vi "Bridge Bias Get Capabilities.vi"(8 "error in":errorcluster, 11 "bridge in":T1={"type"=enum."TWM client", "TWM"={"pipe name"="", "parameters"=[], "handle"=0, "fixed aper [s]"=0.0, "f-list [Hz]"=[], "discrete f-list"=FALSE, "unc mode"=enum."None", "unc mcc"=0, "unc first"=FALSE}, "last f"=0.0, "bias comp"={"bias type"=enum."dummy", "VISA"="", "Enable"=FALSE, "channel qu"=[], "channel Uinit"=[]}, "sim mode"=enum."Generic RLC network", "channel idns"=[], "sim phases"=1} {"TWM"."f-list [Hz]" format="%#_6p"}) -> (0 "error out":errorcluster, 1 "channels count":i32, 2 "max. level [V]":dbl, 3 "bridge out":T1={"type"=enum."TWM client", "TWM"={"pipe name"="", "parameters"=[], "handle"=0, "fixed aper [s]"=0.0, "f-list [Hz]"=[], "discrete f-list"=FALSE, "unc mode"=enum."None", "unc mcc"=0, "unc first"=FALSE}, "last f"=0.0, "bias comp"={"bias type"=enum."dummy", "VISA"="", "Enable"=FALSE, "channel qu"=[], "channel Uinit"=[]}, "sim mode"=enum."Generic RLC network", "channel idns"=[], "sim phases"=1} {"TWM"."f-list [Hz]" format="%#_6p"})   [LabVIEW 2020]
doc: "Get basic capabilities of DC bias compensator."
uses:
  Bridge Session.ctl
  Bridge Type.ctl
  drivers/TWM client/TWM Session.ctl
  drivers/TWM client/TWM parameters.ctl
  drivers/TWM client/Meas Proc QWTB Uncertainty Mode.ctl
  Bridge Bias Session.ctl
  Bridge Bias Type.ctl
  Bridge Sim Mode.ctl
  <vilib>/Utility/error.llb/Error Cluster From Error Code.vi
  <vilib>/ErrorRing/Error Ring.xnode
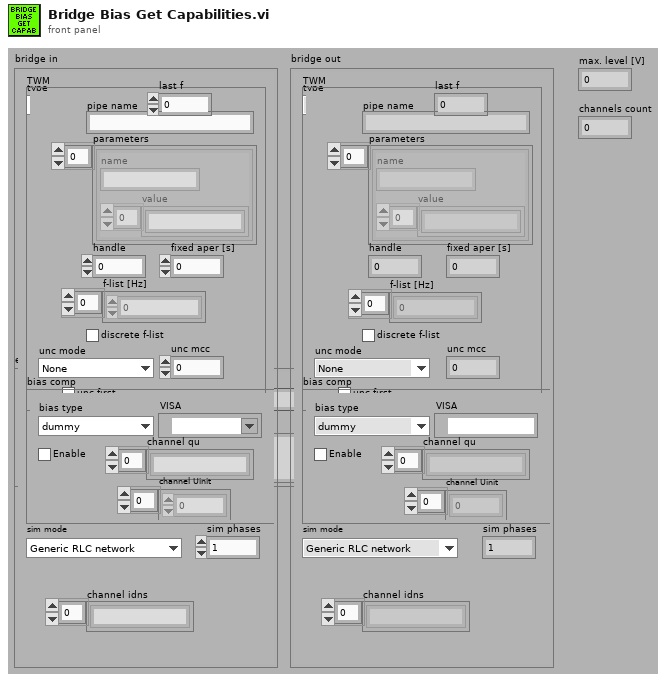
[diagram p1: front panel]
types:
  T1 = typedef "Bridge Session.ctl" = cluster{"type":T2, "TWM":T3, "last f":dbl, "bias comp":T6, "sim mode":T8, "channel idns":string[], "sim phases":i32}
  T2 = typedef "Bridge Type.ctl" = enum16{"TWM client", "dummy"}
  T3 = typedef "TWM Session.ctl" = cluster{"pipe name":string, "parameters":T4[], "handle":i32, "fixed aper [s]":dbl, "f-list [Hz]":dbl[], "discrete f-list":bool, "unc mode":T5, "unc mcc":i32, "unc first":bool}
  T4 = typedef "TWM parameters.ctl" = cluster{"name":string, "value":string[]}
  T5 = typedef "Meas Proc QWTB Uncertainty Mode.ctl" = enum16{"None", "GUF", "Monte Carlo"}
  T6 = typedef "Bridge Bias Session.ctl" = cluster{"bias type":T7, "VISA":refnum<visa-resource-name>, "Enable":bool, "channel qu":string[], "channel Uinit":dbl[]}
  T7 = typedef "Bridge Bias Type.ctl" = enum16{"dummy", "CMI LiBbias V1.0"}
  T8 = typedef "Bridge Sim Mode.ctl" = enum16{"Generic RLC network", "Interchannel transfer"}
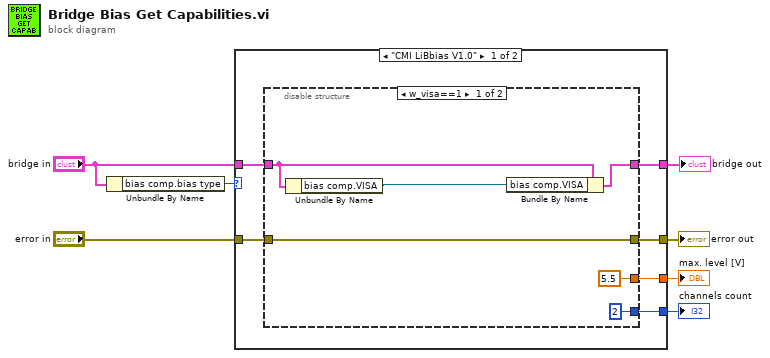
[diagram p0: block diagram]
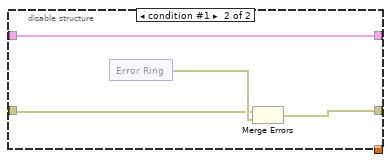
[diagram p2: hidden frame]
diagram:
  n1 = Unbundle By Name("bridge in") -> ("bias comp.bias type"=w7:T7)
  n2 = case shown="\"CMI LiBbias V1.0\"" w7 {
    tunnel: "error in" -> [w11 w30]
    tunnel: [w10 w30] -> w5
    tunnel: "bridge in" -> [w13 w29]
    tunnel: [w12 w29] -> w3
    tunnel: [w9 _] -> w2
    tunnel: [w8 _] -> w1
    frame "CMI LiBbias V1.0" {
      n3 = disable-structure shown="w_visa==1" {
        disable-tunnel: w13 -> [w19 w20]
        disable-tunnel: [w18 w20] -> w12
        disable-tunnel: w11 -> [w16 w22]
        disable-tunnel: [w16 w21] -> w10
        disable-tunnel: [5.5 _] -> w9
        disable-tunnel: [2 ("channels count") _] -> w8
        frame condition #0 (active) {
          n4 = Unbundle By Name(w19) -> ("bias comp.VISA"=w17:refnum<visa-resource-name>)
          n5 = Bundle By Name(cluster=w19, "bias comp.VISA"=w17) -> (w18:T1)
        }
        frame condition #1 {
          n6 = xnode "Error Ring"() -> ("error out"=w23:errorcluster)
          n7 = Merge Errors(w22, w23) -> (w21:errorcluster)
        }
      }
    }
    frame Default {
    }
  }
  "error out" <- w5
  "bridge out" <- w3
  "max. level [V]" <- w2
  "channels count" <- w1
